vi "1Darray rotation.vi"() -> ()   [LabVIEW 2024]
panel:
  in  "Delay":dbl
  out "Reversed Array":bool[](array[boolean])
  out "Bollean Array":bool[](array[boolean])
  out "Rotated Array":dbl[](array[numeric])
  in  "Array":dbl[](array[numeric])
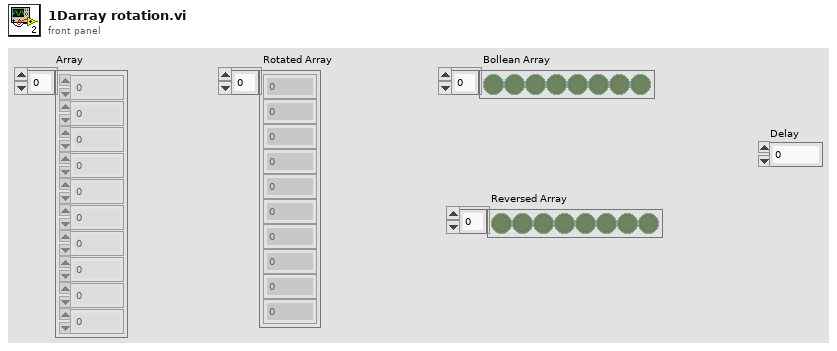
[diagram p1: front panel]
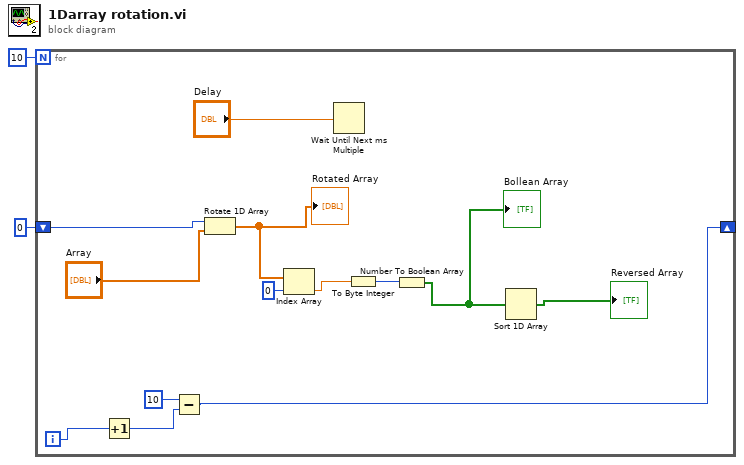
[diagram p0: block diagram]
diagram:
  n1 = for {
    N: 10 -> [_]
    shift-right: [w9] -> _
    shift-left: 0 -> [w15]
    i -> [w12]
    n2 = Increment(x=w12) -> (x+1=w11:i32)
    n3 = Subtract(x=10, y=w11) -> (x-y=w9:i32)
    n4 = Rotate 1D Array(1:"Array", 2:w15) -> (0:w8:dbl[])
    "Rotated Array" <- w8
    n5 = Index Array(array=w8, index=0) -> (element=w6:dbl)
    n6 = Wait Until Next ms Multiple(millisecond multiple="Delay") -> ()  [unwired: 1 out]
    n7 = To Byte Integer(number=w6) -> (8bit integer=w5:i8)
    n8 = Number To Boolean Array(number=w5) -> (Boolean array=w3:bool[])
    "Bollean Array" <- w3
    n9 = Sort 1D Array(array=w3) -> (sorted array=→"Reversed Array":bool[])
  }
